vi "Initialize Phone Number.vi"(8 "error in (no error)":errorcluster, 9 "Region":T1, 10 "Phone Number":string, 11 "AWS Credentials":T2) -> (0 "error out":errorcluster, 3 "Phone Number":refnum<class "Phone Number.lvclass">)   [LabVIEW 2015, in "NI_AWS_SNS.lvlib" / "Phone Number.lvclass"]
doc: "Returns the requested phone number object."
uses:
  Phone Number.lvclass
  Core/HTTP Request/AWS Credentials.ctl
  Core/HTTP Request/Region.ctl
  Core/HTTP Request/Valid String Specification.ctl
  Core/HTTP Request/HTTP Request.lvclass/HTTP Request.ctl
  Phone Number.lvclass/Phone Number.ctl
  Core/HTTP Request/Write Credentials.vi
  Core/HTTP Request/Write Region.vi
  Core/HTTP Request/Write Service.vi
  Core/HTTP Request/Write Verify Server.vi
  Write Phone Number.vi
  Core/HTTP Request/HTTP Request.lvclass
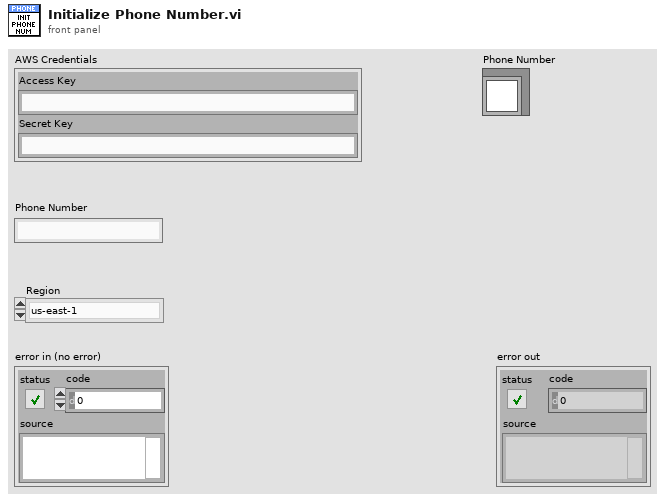
[diagram p1: front panel]
types:
  T1 = typedef "NI_AWS_Core.lvlib/HTTP Request.lvclass/Region.ctl" = enum16{"us-east-1", "us-east-2", "us-west-1", "us-west-2", "ap-northeast-1", "ap-northeast-2", "ap-southeast-1", "ap-southeast-2", "ca-central-1", "eu-central-1", "eu-west-1", "eu-west-2", "sa-east-1"}
  T2 = typedef "NI_AWS_Core.lvlib/HTTP Request.lvclass/AWS Credentials.ctl" = cluster{"Access Key":string, "Secret Key":string}
  T3 = typedef "NI_AWS_Core.lvlib/HTTP Request.lvclass/Valid String Specification.ctl" = enum16{"only [alphanumeric][-][_]", "phone number +1xxxyyyzzzz"}
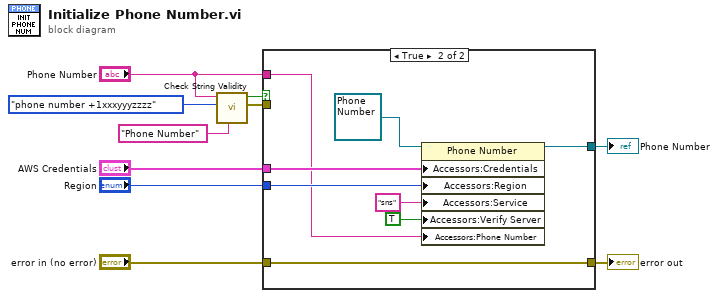
[diagram p0: block diagram]
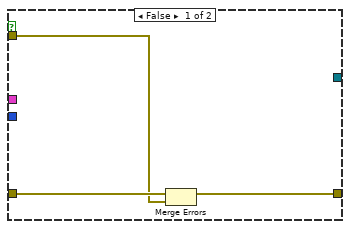
[diagram p2: hidden frame]
diagram:
  n1 = call "Check String Validity.vi"("String Name for Error"="Phone Number", "Valid String Specification"=Valid_String_Specification."phone number +1xxxyyyzzzz", "String"="Phone Number") -> ("string error"=w4:errorcluster, "Valid"=w5:bool)  [unwired: 7 in]
  n2 = case shown="True" w5 {
    tunnel: "AWS Credentials" -> [_ w19]
    tunnel: "error in (no error)" -> [w13 w17]
    tunnel: "Region" -> [_ w16]
    tunnel: [w12 w17] -> w7
    tunnel: [_ w14] -> w6
    tunnel: "Phone Number" -> [_ w15]
    tunnel: w4 -> [w11 _]
    frame False {
      n3 = Merge Errors(w13, w11) -> (w12:errorcluster)
    }
    frame True {
      n4 = property class="Phone Number"(reference=refnum<class "Phone Number.lvclass"> refnum ("NI_AWS_SNS.lvlib:Phone Number.lvclass"), "Accessors:Credentials"=w19, "Accessors:Region"=w16, "Accessors:Service"="sns" ("Service"), "Accessors:Verify Server"=TRUE ("Verify Server"), "Accessors:Phone Number"=w15) -> (reference out=w14:refnum<class "Phone Number.lvclass">)  [unwired: 1 in, 1 out]
    }
  }
  "error out" <- w7
  "Phone Number" <- w6
